vi "set_tasks.vi"(8 "error in (no error)":errorcluster, 9 "counter tasks":refnum<k21>[](array[refnum]), 10 "output tasks":refnum<k21>[](array[refnum]), 11 "DAQmxWriteSignals in":refnum<class "SignalWriterMM140725DAQmx.lvclass">) -> (0 "error out":errorcluster, 3 "DAQmxWriteSignals out":refnum<class "SignalWriterMM140725DAQmx.lvclass">)   [LabVIEW 2010, in "SignalWriterMM140725DAQmx.lvclass"]
uses:
  SignalWriterMM140725DAQmx.lvclass
  class_data.vi
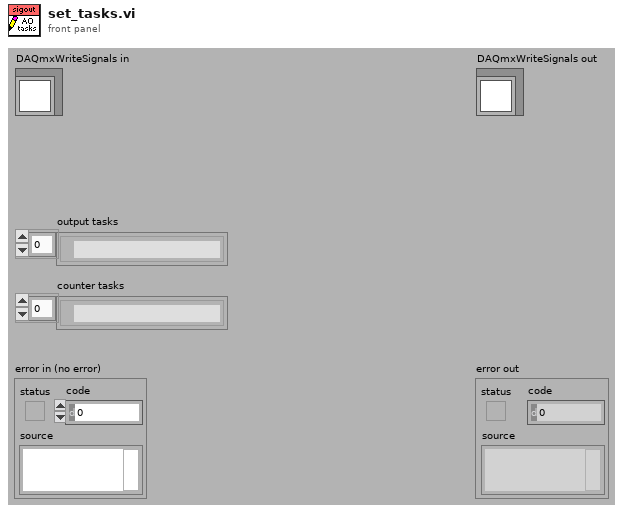
[diagram p1: front panel]
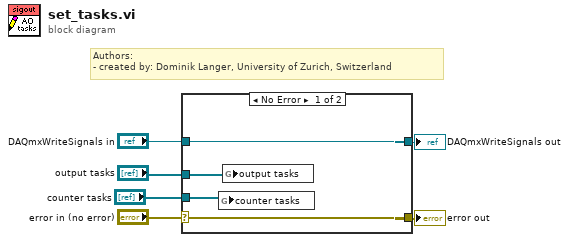
[diagram p0: block diagram]
diagram:
  # "Authors: \n- created by: Dominik Langer, University of Zurich, Switzerland"
  n1 = case shown="No Error" "error in (no error)" {
    selector: "error in (no error)" -> [w9 w12]
    tunnel: [w9 w12] -> w5
    tunnel: [w10 w11] -> w3
    tunnel: "DAQmxWriteSignals in" -> [w10 w11]
    tunnel: "output tasks" -> [w8 _]
    tunnel: "counter tasks" -> [w7 _]
    frame No Error {
      n2 = global write "class_data.vi" "counter tasks"(w7) -> ()
      n3 = global write "class_data.vi" "output tasks"(w8) -> ()
    }
    frame Error {
    }
  }
  "error out" <- w5
  "DAQmxWriteSignals out" <- w3
